vi "S2C_FORNAX_Proc_SendViper.vi"(8 "Error In":errorcluster, 11 "Q-Ref":refnum<queue>) -> (0 "Error Out":errorcluster)   [LabVIEW 2015]
uses:
  S2C_FORNAX_Proc_Globals.vi
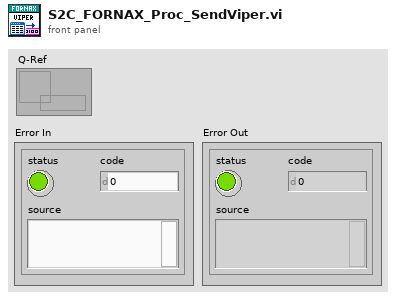
[diagram p1: front panel]
types:
  T1 = cluster{"Caller-Q":refnum<queue>, "Command":string, "Return":string, "Data":variant, "Timeout":dbl}
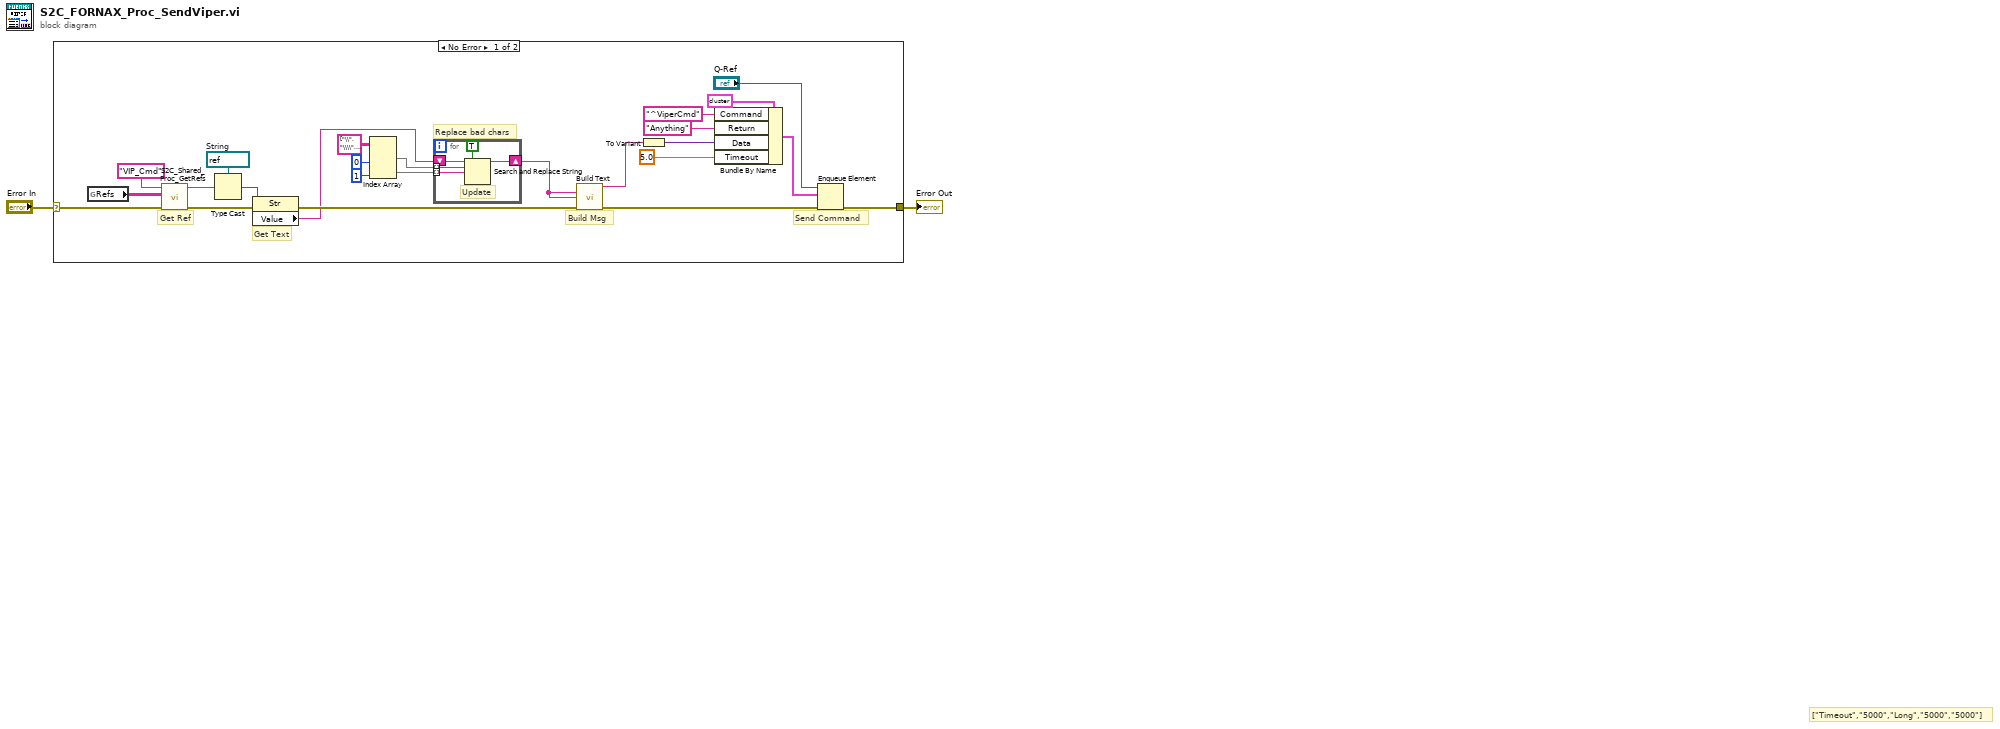
[diagram p0: block diagram]
diagram:
  # "[\"Timeout\",\"5000\",\"Long\",\"5000\",\"5000\"]"
  n1 = case shown="No Error" "Error In" {
    selector: "Error In" -> [w14 w33]
    tunnel: [w25 w33] -> w1
    frame No Error {
      w22 = refnum<vi> refnum  # String
      # "Get Text"
      # "Replace bad chars"
      # "Build Msg"
      # "Get Ref"
      # "Send Command"
      n2 = global read "S2C_FORNAX_Proc_Globals.vi" "Refs"() -> (w17:string[][])
      n3 = call "S2C_Shared_Proc_GetRefs.vi"("Error In"=w14, "Refs"=w17, "Label"="VIP_Cmd") -> ("Error Out"=w23:errorcluster, "Reference"=w21:string)  [unwired: 7 in]
      n4 = Type Cast(type=w22, x=w21) -> (*(type *) &x=w20:refnum<vi>)
      n5 = property class="Str"(reference=w20, error in=w23) -> (error out=w7:errorcluster, "Value"=w4:string)  [unwired: 1 out]
      n6 = Index Array(array=string[][] [["\\", "\\\\"], ["\"", "\\\""], ["\n", "\\n"], ["\r", "\\r"], ["\t", "\\t"]], index (col) #1=0 ("disabled index (col)"), index (col) #2=1 ("index (col)")) -> (element #1=w11:string[], element #2=w12:string[])  [unwired: 2 in]
      n7 = for {
        tunnel: w11 -> [w31] mode=indexing
        tunnel: w12 -> [w29] mode=indexing
        shift-right: [w28] -> w3
        shift-left: w4 -> [w32]
        # "Update"
        n8 = Search and Replace String(replace all?=TRUE ("replace all? (F)"), input string=w32, search string=w31, replace string=w29) -> (result string=w28:string)  [unwired: 4 in, 3 out]
      }
      n9 = call "Build Text"("Msg"=w3, "Msg1"=w3, "error in (no error)"=w7) -> ("Result"=w6:string, "error out"=w5:errorcluster)  [unwired: 11 in]
      n10 = To Variant(anything=w6) -> (Variant=w18:variant)
      n11 = Bundle By Name(cluster=T1 {"Caller-Q"=refnum, "Command"="", "Return"="None", "Data"=variant, "Timeout"=10.0} ("element"), "Command"="^ViperCmd" ("string"), "Return"="Anything", "Data"=w18, "Timeout"=5.0) -> (w24:T1)
      n12 = Enqueue Element(queue="Q-Ref", element=w24, error in (no error)=w5) -> (error out=w25:errorcluster)  [unwired: 1 in, 2 out]
    }
    frame Error {
    }
  }
  "Error Out" <- w1
